vi "Main.vi"() -> ()   [LabVIEW 2022 SP3]
doc: "This Continuous Measurement sample project is based on the Queued Message Handler template.\n\nThe Event Handling Loop generates messages based on user interface actions.\n\nThe Message Handling Loop processes messages generated by the Event Handling Loop, or by other messages. There are also Acquisition and Logging message handling loop subVIs, and a chart updating loop."
uses:
  Settings/Settings.ctl
  Logging/Logging Configuration.ctl
  FiniteMeasurement-DAQmx/controls/Hardware Configuration.ctl
  controls/UI Data.ctl
  controls/UI State.ctl
  Logging/LoggedData.ctl
  support/Message Queue/Enqueue Message (Single).vi
  <vilib>/Utility/error.llb/Error Cluster From Error Code.vi
  <vilib>/ErrorRing/Error Ring.xnode
  Acquisition/Acquisition.lvlib
  Logging/Logging.lvlib
  Settings/Settings.lvlib
  support/User Event - Stop/User Event - Stop.lvlib
  support/Message Queue/Message Queue.lvlib
panel:
  out "FFT- Phase":cluster{dbl, dbl, dbl[]}(graph)
  out "FFT- Mag":cluster{dbl, dbl, dbl[]}(graph)
  in  "Block Size":i32=4096
  in  "Output Settings":bool
  in  "Start Output":bool
  in  "Controller Settings":bool
  in  "Start Controller":bool
  in  "Exit":bool
  in  "Settings":bool
  in  "Start":bool
  in  "Force Trigger":bool
  in  "Stop":bool
  in  "Snapshot":bool
  in  "Analyze":bool
  in  "Clear":bool
  in  "Export":bool
  in  "Save Data":bool
  in  "Load Data":bool
  out "Raw":waveform(dbl)[](graph)
  out "Status":string
  # "Continuous Measurement and Logging (NI-DAQmx)"
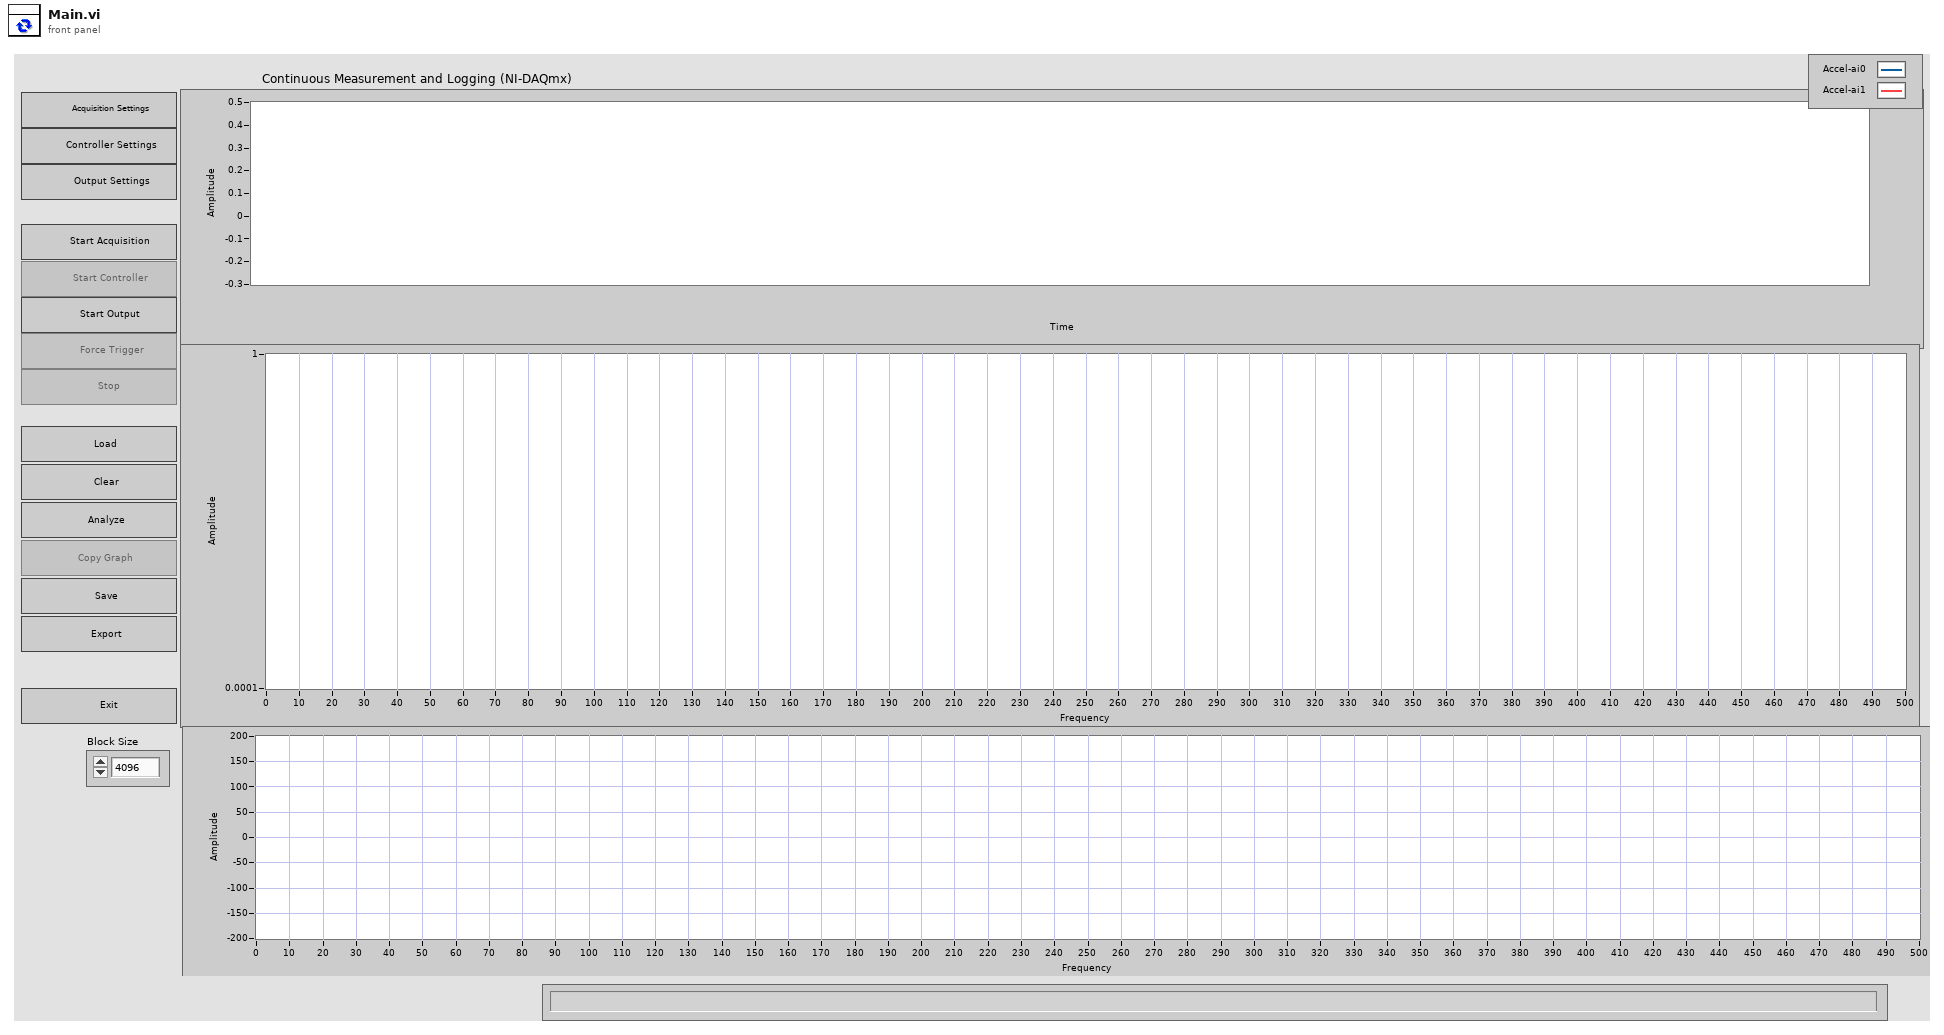
[diagram p1: front panel]
types:
  T1 = typedef "LoggedData.ctl" = cluster{"WaveformArray":waveform(dbl)[], "FFTArray":cluster{dbl, dbl, dbl[]}[]}
  T2 = typedef "UI State.ctl" = enum16{"Idle", "Acquiring and Logging", "Waiting for Exit", "Waiting for Exit (Acq Stopped)", "Waiting for Exit (Log Stopped)", "Waiting for Stop", "Waiting for Stop (Acq Stopped)", "Waiting for Stop (Log Stopped)"}
  T3 = typedef "UI Data.ctl" = cluster{"Start Ref":refnum<vi>, "Trigger Ref":refnum<vi>, "Stop Ref":refnum<vi>, "Settings Ref":refnum<vi>, "Status Ref":refnum<vi>, "Exit Ref":refnum<vi>, "Data Ref":refnum<vi>, "Clear Ref":refnum<vi>, "Load Data Ref":refnum<vi>, "Analyse Ref":refnum<vi>, "Snapshot Ref":refnum<vi>, "Save Data Ref":refnum<vi>, "Export Ref":refnum<vi>, "Output Setting Ref":refnum<vi>, "Start Output Ref":refnum<vi>, "Controller Settings Ref":refnum<vi>, "Start Controller Ref":refnum<vi>}
  T4 = typedef "Settings.lvlib/Settings.ctl" = cluster{"Logging Configuration":T5, "Hardware Configuration":T6}
  T5 = typedef "Logging.lvlib/Logging Configuration.ctl" = cluster{"Log File Base Path":path, "TDMS File Reference":refnum<k34>, "Samples to Save":u32, "Trigger - Time":u32, "Trigger - Threshold":dbl, "Trigger - Channel":u32, "Enable Time Trigger":bool, "Enable Threshold Trigger":bool, "Always Log":bool}
  T6 = typedef "Acquisition.lvlib/Hardware Configuration.ctl" = cluster{"Accel-ai0":bool, "Maximum Input":dbl, "Minimum Input":dbl, "Sample Rate":dbl, "Number of Samples":i32, "Accel-ai1":bool, "DAQmx Task":refnum<k21>}
  T7 = typedef "Message Queue.lvlib/All Message Queues.ctl" = cluster{"UI":refnum<queue>, "Acquisition":refnum<queue>, "Logging":refnum<queue>}
  T8 = enum8{"Enabled", "Disabled", "Disabled and Grayed Out"}
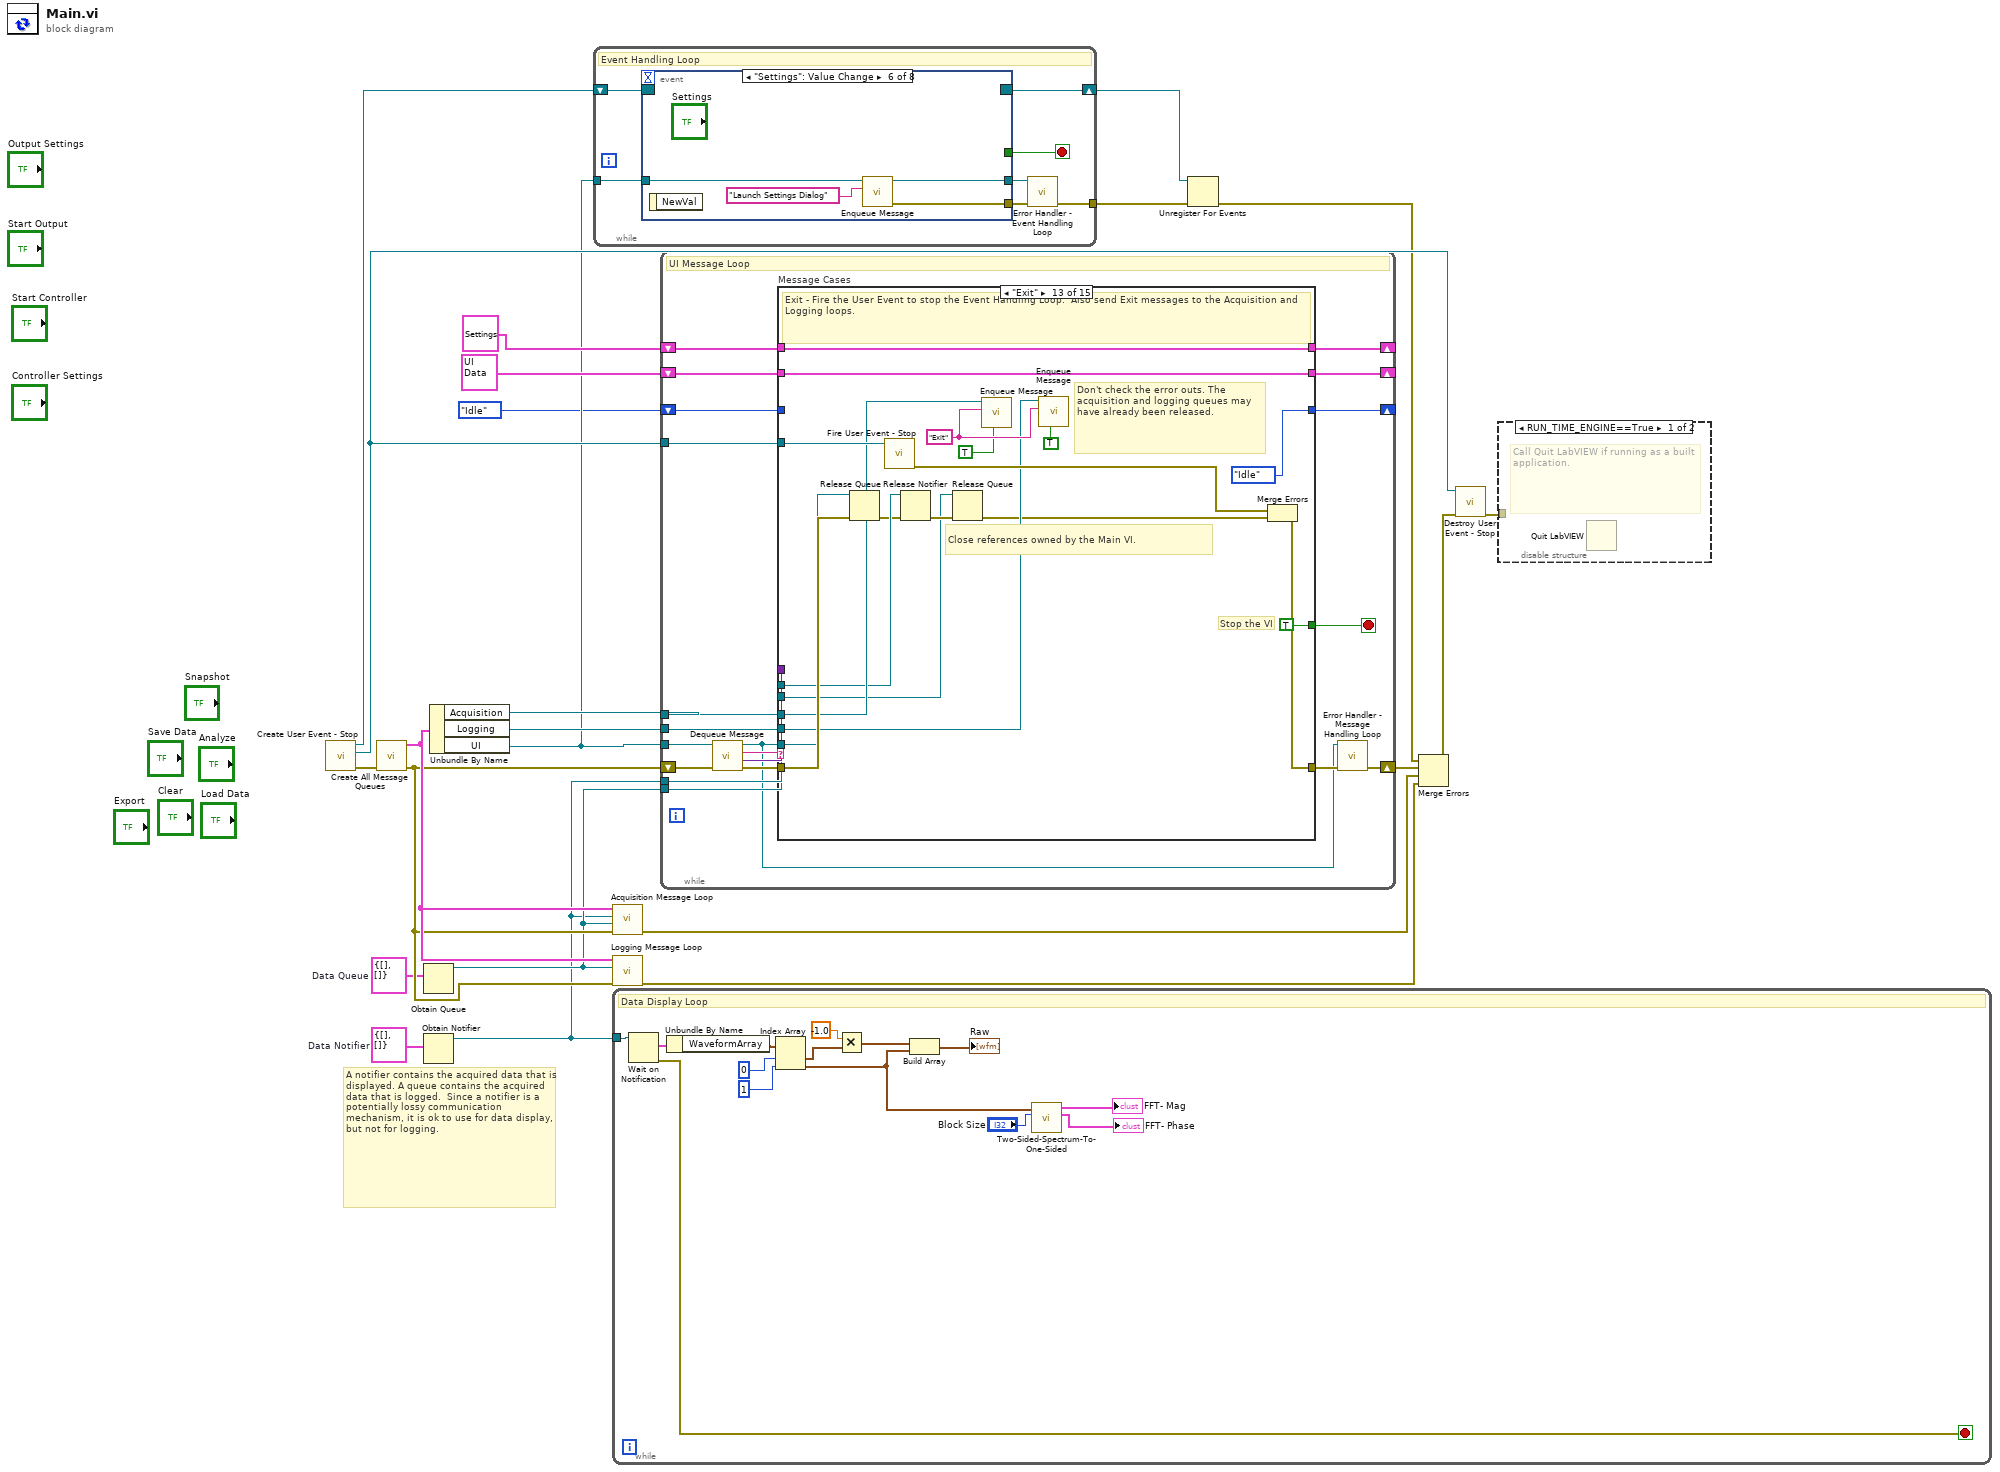
[diagram p0: block diagram]
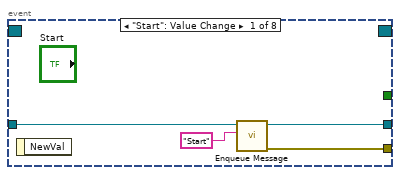
[diagram p3: hidden frame]
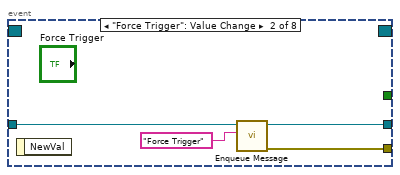
[diagram p4: hidden frame]
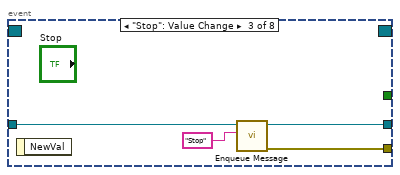
[diagram p5: hidden frame]
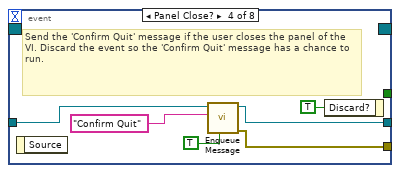
[diagram p6: hidden frame]
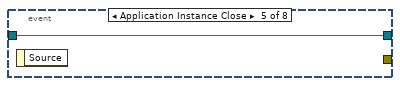
[diagram p7: hidden frame]
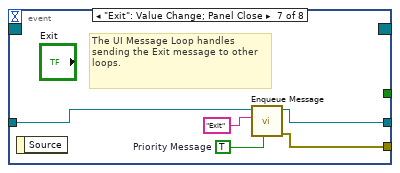
[diagram p8: hidden frame]
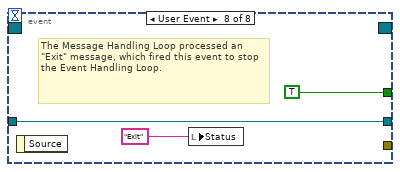
[diagram p9: hidden frame]
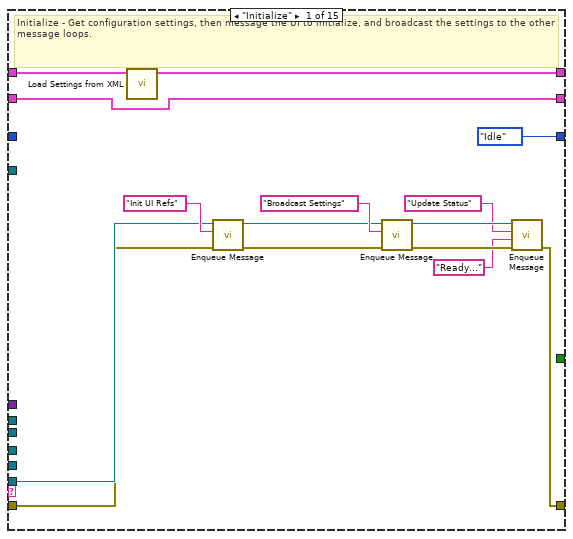
[diagram p10: hidden frame]
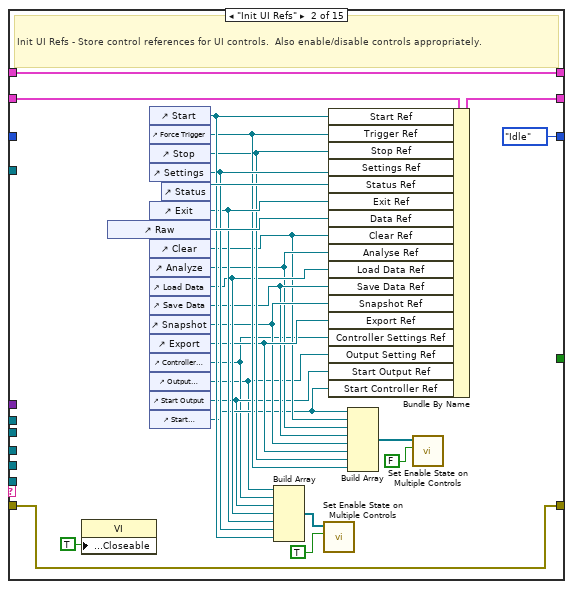
[diagram p11: hidden frame]
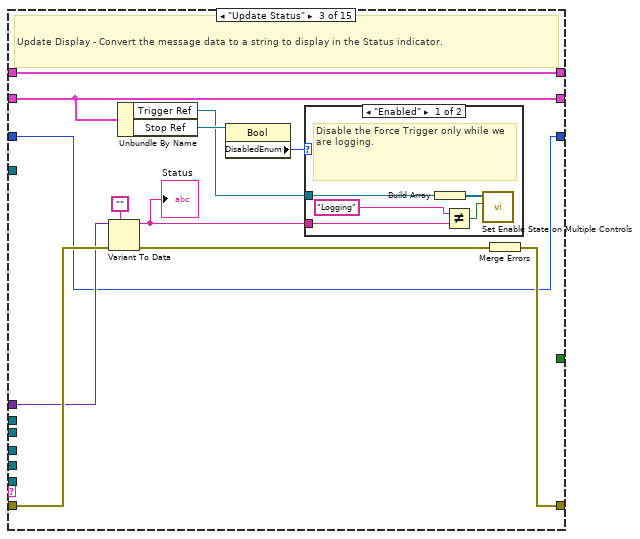
[diagram p12: hidden frame]
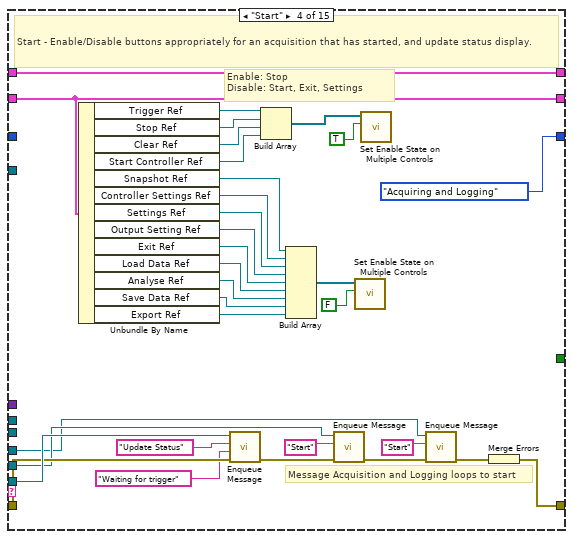
[diagram p14: hidden frame]
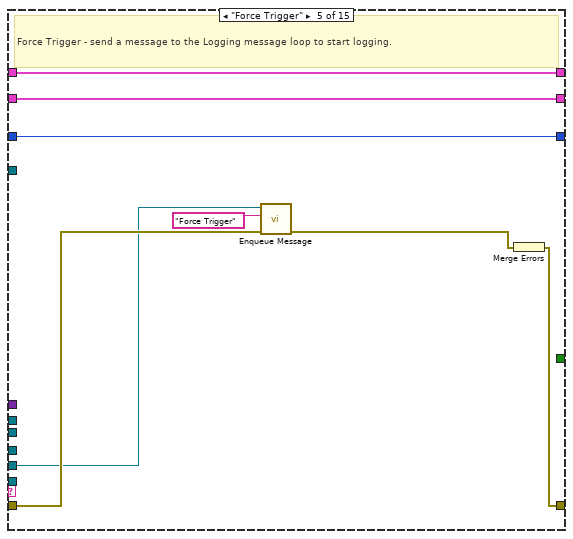
[diagram p15: hidden frame]
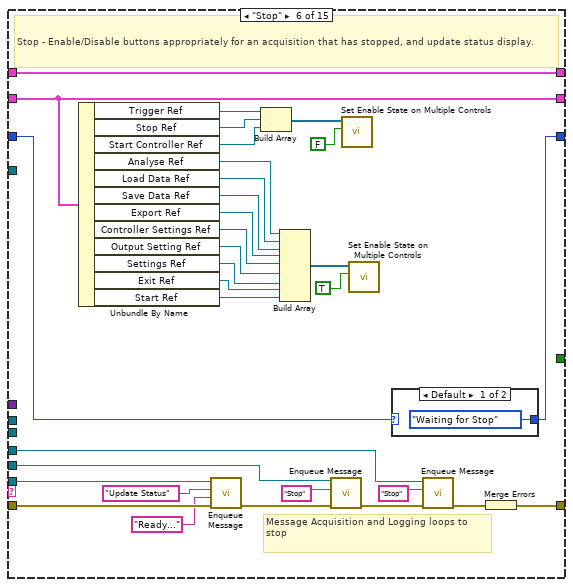
[diagram p16: hidden frame]
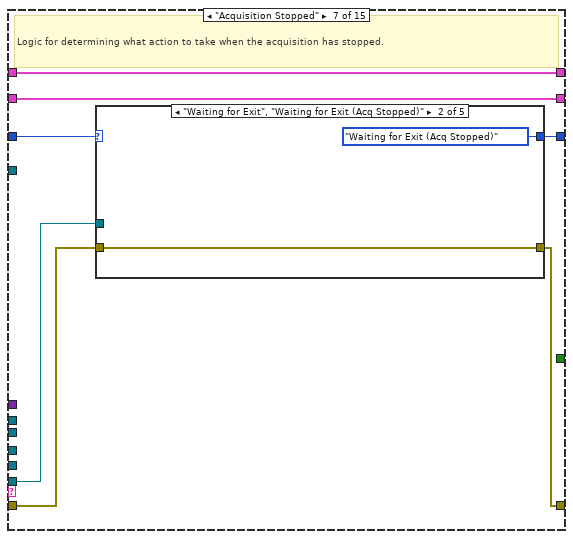
[diagram p18: hidden frame]
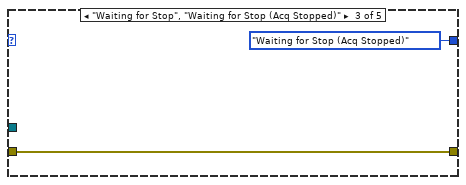
[diagram p20: hidden frame]
diagram:
  w3 = T1 {"WaveformArray"=[], "FFTArray"=[]}  # Data Notifier
  w4 = T1 {"WaveformArray"=[], "FFTArray"=[]}  # Data Queue
  # "A notifier contains the acquired data that is displayed. A queue contains the acquired data that is logged.  Since a notifier is a potentially lossy communication mechanism, it is ok to use for data display, but not for logging."
  n1 = call "Create User Event - Stop.vi"() -> ("error out"=w17:errorcluster, "User Event - Stop"=w19:refnum<user-event>, "Stop Event Registration Refnum"=w20:refnum<event-registration>)  [unwired: 9 in]
  n2 = call "Create All Message Queues.vi"("error in (no error)"=w17) -> ("error out"=w5:errorcluster, "Message Queues out"=w16:T7)  [unwired: 9 in]
  n3 = Obtain Queue(element data type=w4) -> (queue out=w2:refnum<queue>)  [unwired: 4 in, 2 out]
  n4 = Obtain Notifier(notification data type=w3) -> (notifier out=w1:refnum<notifier>)  [unwired: 3 in, 2 out]
  n5 = Unbundle By Name(w16) -> ("Acquisition"=w10:refnum<queue>, "Logging"=w9:refnum<queue>, "UI"=w8:refnum<queue>)
  n6 = while {
    tunnel: w8 -> [w29]
    tunnel: [w24] -> w22
    shift-right: [w28] -> w12
    shift-left: w20 -> [w30]
    stop <- w27 stop-if-true
    # "Event Handling Loop"
    n7 = event shown="[5] \"Settings\": Value Change" {
      selector: w30 -> [_ _ _ _ _ _ _ _]
      dyn-events: [_ _ _ _ _ _ _ _] -> w28
      timeout: _ -> [_ _ _ _ _ _ _ _]
      tunnel: [_ _ _ _ _ _ _ TRUE ("Discard?")] -> w27
      tunnel: w29 -> [w32 w37 w41 w48 w49 w51 w55 w59]
      tunnel: [w34 w36 w40 w43 _ w53 w58 _] -> w25
      tunnel: [w31 w35 w39 w44 w49 w50 w54 w59] -> w26
      event "Start": Value Change {
        n8 = event-data() -> ()  [unwired: 1 in, 1 out]
        n9 = call-poly "Enqueue Message.vi"("Message"="Start", "Message Queue"=w32) -> ("error out"=w34:errorcluster, "dup Message Queue"=w31:refnum<queue>)  [unwired: 8 in]
      }
      event "Force Trigger": Value Change {
        n10 = event-data() -> ()  [unwired: 1 in, 1 out]
        n11 = call-poly "Enqueue Message.vi"("Message"="Force Trigger", "Message Queue"=w37) -> ("error out"=w36:errorcluster, "dup Message Queue"=w35:refnum<queue>)  [unwired: 8 in]
      }
      event "Stop": Value Change {
        n12 = event-data() -> ()  [unwired: 1 in, 1 out]
        n13 = call-poly "Enqueue Message.vi"("Message"="Stop", "Message Queue"=w41) -> ("error out"=w40:errorcluster, "dup Message Queue"=w39:refnum<queue>)  [unwired: 8 in]
      }
      event Panel Close? {
        # "Send the 'Confirm Quit' message if the user closes the panel of the VI. Discard the event so the 'Confirm Quit' message has a chance to run."
        n14 = event-data() -> ()  [unwired: 1 in, 1 out]
        n15 = call-poly "Enqueue Message.vi"("Priority Message? (F)"=TRUE, "Message"="Confirm Quit", "Message Queue"=w48) -> ("error out"=w43:errorcluster, "dup Message Queue"=w44:refnum<queue>)  [unwired: 7 in]
        n16 = event-data("Discard?"=TRUE) -> ()  [unwired: 1 in, 1 out]
      }
      event Application Instance Close {
        n17 = event-data() -> ()  [unwired: 1 in, 1 out]
      }
      event "Settings": Value Change {
        n18 = event-data() -> ()  [unwired: 1 in, 1 out]
        n19 = call-poly "Enqueue Message.vi"("Message"="Launch Settings Dialog", "Message Queue"=w51) -> ("error out"=w53:errorcluster, "dup Message Queue"=w50:refnum<queue>)  [unwired: 8 in]
      }
      event "Exit": Value Change; Panel Close {
        w56 = TRUE  # Priority Message
        # "The UI Message Loop handles sending the Exit message to other loops."
        n20 = event-data() -> ()  [unwired: 1 in, 1 out]
        n21 = call-poly "Enqueue Message.vi"("Priority Message? (F)"=w56, "Message"="Exit", "Message Queue"=w55) -> ("error out"=w58:errorcluster, "dup Message Queue"=w54:refnum<queue>)  [unwired: 7 in]
      }
      event User Event {
        # "The Message Handling Loop processed an \"Exit\" message, which fired this event to stop the Event Handling Loop."
        n22 = event-data() -> ()  [unwired: 1 in, 1 out]
        n23 = local write "Status"("Exit" ("Exit String")) -> ()
      }
    }
    n24 = call "Error Handler - Event Handling Loop.vi"("error in (no error)"=w25, "Message Queue"=w26) -> ("dup error in"=w24:errorcluster)  [unwired: 8 in, 1 out]
  }
  n25 = call "Acquisition Message Loop.vi"("error in (no error)"=w5, "Data Queue"=w2, "Data Notifier"=w1, "Message Queues"=w16) -> ("error out"=w18:errorcluster)  [unwired: 7 in]
  n26 = call "Logging Message Loop.vi"("error in (no error)"=w5, "Data Queue"=w2, "Message Queues"=w16) -> ("error out"=w15:errorcluster)  [unwired: 8 in]
  n27 = while "Data Display Loop" {
    tunnel: w1 -> [w75]
    stop <- w62 stop-if-true
    # "Data Display Loop"
    n28 = Wait on Notification(notifier=w75) -> (notification=w68:T1, error out=w62:errorcluster)  [unwired: 3 in, 2 out]
    n29 = Unbundle By Name(w68) -> ("WaveformArray"=w67:waveform(dbl)[])
    n30 = Index Array(array=w67, index #1=0 ("index"), index #2=1 ("index")) -> (element #1=w70:waveform(dbl), element #2=w66:waveform(dbl))
    n31 = Multiply(x=-1.0, y=w70) -> (x*y=w69:waveform(dbl))
    n32 = Build Array(w69, w66) -> (→"Raw":waveform(dbl)[])
    n33 = call "Two-Sided-Spectrum-To-One-Sided.vi"("Block Size"="Block Size", "waveform"=w66) -> ("FFT- Phase"=→"FFT- Phase":cluster{dbl, dbl, dbl[]}, "FFT- Mag"=→"FFT- Mag":cluster{dbl, dbl, dbl[]})  [unwired: 8 in]
  }
  n34 = while {
    tunnel: w8 -> [w89]
    tunnel: w19 -> [w94]
    shift-right: [w79] -> w23
    shift-left: w5 -> [w93]
    shift-right: [w88] -> _
    shift-left: T4 {"Logging Configuration"={"Log File Base Path"=path "", "TDMS File Reference"=refnum, "Samples to Save"=0, "Trigger - Time"=0, "Trigger - Threshold"=0.0, "Trigger - Channel"=0, "Enable Time Trigger"=FALSE, "Enable Threshold Trigger"=FALSE, "Always Log"=FALSE}, "Hardware Configuration"={"Accel-ai0"=FALSE, "Maximum Input"=0.0, "Minimum Input"=0.0, "Sample Rate"=0.0, "Number of Samples"=0, "Accel-ai1"=FALSE, "DAQmx Task"=""}} ("Settings") -> [w87]
    shift-right: [w85] -> _
    shift-left: T3 {"Start Ref"=refnum, "Trigger Ref"=refnum, "Stop Ref"=refnum, "Settings Ref"=refnum, "Status Ref"=refnum, "Exit Ref"=refnum, "Data Ref"=refnum, "Clear Ref"=refnum, "Load Data Ref"=refnum, "Analyse Ref"=refnum, "Snapshot Ref"=refnum, "Save Data Ref"=refnum, "Export Ref"=refnum, "Output Setting Ref"=refnum, "Start Output Ref"=refnum, "Controller Settings Ref"=refnum, "Start Controller Ref"=refnum} ("Measurement UI Controls") -> [w86]
    tunnel: w10 -> [w84]
    tunnel: w9 -> [w83]
    tunnel: w1 -> [w82]
    tunnel: w2 -> [w81]
    shift-right: [w76] -> _
    shift-left: UI_State."Idle" ("UI State") -> [w77]
    stop <- w95 stop-if-true
    # "UI Message Loop"
    n35 = call "Dequeue Message.vi"("error in (no error)"=w93, "Message Queue"=w89) -> ("error out"=w92:errorcluster, "Message Data"=w90:variant, "Message"=w91:string, "dup Message Queue"=w78:refnum<queue>)  [unwired: 6 in]
    n36 = case "Message Cases" shown="\"Exit\"" w91 {
      selector: w91 -> [_ _ _ _ _ _ _ _ _ _ _ _ _ _ w371]
      tunnel: w78 -> [w100 _ _ w185 _ w225 w229 w254 _ w296 w311 w321 w354 _ _]
      tunnel: w92 -> [w99 w137 w148 w184 w191 w224 w231 w256 w284 w298 w315 w320 w362 w369 _]
      tunnel: [w106 w137 w149 w186 w194 w226 w230 w255 w290 w293 w306 w319 w363 w368 w372] -> w80
      tunnel: [_ _ _ _ _ _ _ _ _ _ _ _ TRUE _ _] -> w95
      tunnel: w90 -> [_ _ w147 _ _ _ _ _ _ _ w314 _ _ _ _]
      tunnel: w94 -> [_ _ _ _ _ _ _ _ _ _ _ _ w361 _ _]
      tunnel: [w109 w136 w144 w183 w193 w223 w235 w260 w288 w295 w317 w324 w359 w367 w374] -> w88
      tunnel: w87 -> [w110 w136 w144 w183 w193 w223 w235 w260 w288 w299 w317 w324 w359 w367 w374]
      tunnel: w86 -> [w102 w135 w143 w180 w192 w220 w234 w259 w282 w292 w316 w323 w357 w366 w373]
      tunnel: [w102 w134 w143 w180 w192 w220 w234 w259 w282 w292 w316 w323 w357 w366 w373] -> w85
      tunnel: w84 -> [_ _ _ w170 _ w210 _ _ w281 _ _ _ w356 _ _]
      tunnel: w83 -> [_ _ _ w173 w188 w213 _ _ w280 _ _ _ w355 _ _]
      tunnel: w82 -> [_ _ _ _ _ _ _ _ _ _ _ _ w353 _ _]
      tunnel: w81 -> [_ _ _ _ _ _ _ _ _ _ _ _ w349 _ _]
      tunnel: w77 -> [_ _ w138 _ w187 w206 w233 w258 w279 w291 w305 w322 _ w365 w370]
      tunnel: [UI_State."Idle" ("UI State") UI_State."Idle" ("UI State") w138 UI_State."Acquiring and Logging" ("UI State") w187 w205 w232 w257 w279 w291 w305 w318 UI_State."Idle" ("UI State") w365 w370] -> w76
      frame "Initialize" {
        # "Initialize - Get configuration settings, then message the UI to initialize, and broadcast the settings to the other message loops."
        n37 = call "Load Settings from XML.vi"("Settings in"=w110) -> ("Settings out"=w109:T4)  [unwired: 9 in, 1 out]
        n38 = call-poly "Enqueue Message.vi"("error in (no error)"=w99, "Message"="Init UI Refs", "Message Queue"=w100) -> ("error out"=w97:errorcluster, "dup Message Queue"=w98:refnum<queue>)  [unwired: 7 in]
        n39 = call-poly "Enqueue Message.vi"("error in (no error)"=w97, "Message"="Broadcast Settings", "Message Queue"=w98) -> ("error out"=w108:errorcluster, "dup Message Queue"=w107:refnum<queue>)  [unwired: 7 in]
        n40 = call-poly "Enqueue Message.vi"("error in (no error)"=w108, "Message Data"="Ready..." ("Ready..."), "Message"="Update Status", "Message Queue"=w107) -> ("error out"=w106:errorcluster)  [unwired: 6 in, 1 out]
      }
      frame "Init UI Refs" {
        # "Init UI Refs - Store control references for UI controls.  Also enable/disable controls appropriately."
        n41 = property class="VI"("Front Panel.Closeable"=TRUE ("Front Panel Window:Closeable")) -> ()  [unwired: 2 in, 2 out]
        n42 = control-ref of="Raw"() -> (w130:refnum<vi>)
        n43 = control-ref of="Start"() -> (w129:refnum<vi>)
        n44 = control-ref of="Force Trigger"() -> (w124:refnum<vi>)
        n45 = control-ref of="Stop"() -> (w123:refnum<vi>)
        n46 = control-ref of="Settings"() -> (w126:refnum<vi>)
        n47 = control-ref of="Exit"() -> (w125:refnum<vi>)
        n48 = control-ref of="Clear"() -> (w115:refnum<vi>)
        n49 = control-ref of="Analyze"() -> (w116:refnum<vi>)
        n50 = control-ref of="Load Data"() -> (w120:refnum<vi>)
        n51 = control-ref of="Save Data"() -> (w117:refnum<vi>)
        n52 = control-ref of="Snapshot"() -> (w118:refnum<vi>)
        n53 = control-ref of="Export"() -> (w119:refnum<vi>)
        n54 = control-ref of="Controller Settings"() -> (w112:refnum<vi>)
        n55 = control-ref of="Output Settings"() -> (w111:refnum<vi>)
        n56 = control-ref of="Start Output"() -> (w113:refnum<vi>)
        n57 = control-ref of="Start Controller"() -> (w114:refnum<vi>)
        n58 = control-ref of="Status"() -> (w131:refnum<vi>)
        n59 = Build Array(w111, w112, w113, w120, w125, w126, w129) -> (w128:refnum<vi>[])
        n60 = call "Set Enable State on Multiple Controls.vi"("Enable?"=TRUE, "Controls"=w128) -> ()  [unwired: 10 in]
        n61 = Bundle By Name(cluster=w135, "Start Ref"=w129, "Trigger Ref"=w124, "Stop Ref"=w123, "Settings Ref"=w126, "Status Ref"=w131, "Exit Ref"=w125, "Data Ref"=w130, "Clear Ref"=w115, "Analyse Ref"=w116, "Load Data Ref"=w120, "Save Data Ref"=w117, "Snapshot Ref"=w118, "Export Ref"=w119, "Controller Settings Ref"=w112, "Output Setting Ref"=w111, "Start Output Ref"=w113, "Start Controller Ref"=w114) -> (w134:T3)
        n62 = Build Array(w114, w115, w116, w117, w118, w119, w123, w124) -> (w122:refnum<vi>[])
        n63 = call "Set Enable State on Multiple Controls.vi"("Enable?"=FALSE, "Controls"=w122) -> ()  [unwired: 10 in]
      }
      frame "Update Status" {
        # "Update Display - Convert the message data to a string to display in the Status indicator."
        n64 = Variant To Data(error in=w148, type="", Variant=w147) -> (data=w140:string, error out=w145:errorcluster)
        "Status" <- w140
        n65 = Unbundle By Name(w143) -> ("Trigger Ref"=w139:refnum<vi>, "Stop Ref"=w142:refnum<vi>)
        n66 = property class="Bool"(reference=w142) -> ("DisabledEnum"=w141:T8)  [unwired: 1 in, 2 out]
        n67 = case shown="\"Enabled\"" w141 {
          tunnel: w140 -> [w152 _]
          tunnel: w139 -> [w153 _]
          frame "Enabled" {
            # "Disable the Force Trigger only while we are logging."
            n68 = Build Array(w153) -> (w154:refnum<vi>[])
            n69 = Not Equal?(x="Logging" ("Logging"), y=w152) -> (x != y?=w150:bool)
            n70 = call "Set Enable State on Multiple Controls.vi"("Enable?"=w150, "Controls"=w154) -> ()  [unwired: 10 in]
          }
          frame "Disabled", Default {
          }
        }
        n71 = Merge Errors(w145) -> (w149:errorcluster)
      }
      frame "Start" {
        # "Message Acquisition and Logging loops to start"
        # "Enable: Stop\nDisable: Start, Exit, Settings"
        # "Start - Enable/Disable buttons appropriately for an acquisition that has started, and update status display."
        n72 = Unbundle By Name(w180) -> ("Trigger Ref"=w167:refnum<vi>, "Stop Ref"=w168:refnum<vi>, "Clear Ref"=w165:refnum<vi>, "Start Controller Ref"=w164:refnum<vi>, "Snapshot Ref"=w155:refnum<vi>, "Controller Settings Ref"=w156:refnum<vi>, "Settings Ref"=w157:refnum<vi>, "Output Setting Ref"=w158:refnum<vi>, "Exit Ref"=w159:refnum<vi>, "Load Data Ref"=w160:refnum<vi>, "Analyse Ref"=w161:refnum<vi>, "Save Data Ref"=w162:refnum<vi>, "Export Ref"=w163:refnum<vi>)
        n73 = call-poly "Enqueue Message.vi"("error in (no error)"=w184, "Message Data"="Waiting for trigger" ("Waiting for trigger"), "Message"="Update Status", "Message Queue"=w185) -> ("error out"=w175:errorcluster)  [unwired: 6 in, 1 out]
        n74 = Build Array(w167, w168, w165, w164) -> (w177:refnum<vi>[])
        n75 = Build Array(w155, w156, w157, w158, w159, w160, w161, w162, w163) -> (w178:refnum<vi>[])
        n76 = call-poly "Enqueue Message.vi"("error in (no error)"=w175, "Message"="Start", "Message Queue"=w173) -> ("error out"=w172:errorcluster)  [unwired: 7 in, 1 out]
        n77 = call "Set Enable State on Multiple Controls.vi"("Enable?"=FALSE, "Controls"=w178) -> ()  [unwired: 10 in]
        n78 = call "Set Enable State on Multiple Controls.vi"("Enable?"=TRUE, "Controls"=w177) -> ()  [unwired: 10 in]
        n79 = call-poly "Enqueue Message.vi"("error in (no error)"=w172, "Message"="Start", "Message Queue"=w170) -> ("error out"=w171:errorcluster)  [unwired: 7 in, 1 out]
        n80 = Merge Errors(w171) -> (w186:errorcluster)
      }
      frame "Force Trigger" {
        # "Force Trigger - send a message to the Logging message loop to start logging."
        n81 = call-poly "Enqueue Message.vi"("error in (no error)"=w191, "Message"="Force Trigger", "Message Queue"=w188) -> ("error out"=w190:errorcluster)  [unwired: 7 in, 1 out]
        n82 = Merge Errors(w190) -> (w194:errorcluster)
      }
      frame "Stop" {
        # "Message Acquisition and Logging loops to stop"
        # "Stop - Enable/Disable buttons appropriately for an acquisition that has stopped, and update status display."
        n83 = Unbundle By Name(w220) -> ("Trigger Ref"=w207:refnum<vi>, "Stop Ref"=w208:refnum<vi>, "Start Controller Ref"=w204:refnum<vi>, "Analyse Ref"=w195:refnum<vi>, "Load Data Ref"=w196:refnum<vi>, "Save Data Ref"=w197:refnum<vi>, "Export Ref"=w198:refnum<vi>, "Controller Settings Ref"=w199:refnum<vi>, "Output Setting Ref"=w200:refnum<vi>, "Settings Ref"=w201:refnum<vi>, "Exit Ref"=w202:refnum<vi>, "Start Ref"=w203:refnum<vi>)
        n84 = call-poly "Enqueue Message.vi"("error in (no error)"=w224, "Message Data"="Ready..." ("Ready..."), "Message"="Update Status", "Message Queue"=w225) -> ("error out"=w215:errorcluster)  [unwired: 6 in, 1 out]
        n85 = Build Array(w207, w208, w204) -> (w217:refnum<vi>[])
        n86 = Build Array(w195, w196, w197, w198, w199, w200, w201, w202, w203) -> (w218:refnum<vi>[])
        n87 = call-poly "Enqueue Message.vi"("error in (no error)"=w215, "Message"="Stop", "Message Queue"=w213) -> ("error out"=w212:errorcluster)  [unwired: 7 in, 1 out]
        n88 = call "Set Enable State on Multiple Controls.vi"("Enable?"=FALSE, "Controls"=w217) -> ()  [unwired: 10 in]
        n89 = call "Set Enable State on Multiple Controls.vi"("Enable?"=TRUE, "Controls"=w218) -> ()  [unwired: 10 in]
        n90 = case shown="Default" w206 {
          selector: w206 -> [_ w228]
          tunnel: [UI_State."Waiting for Stop" ("UI State") w228] -> w205
          frame Default {
          }
          frame "Waiting for Exit" {
          }
        }
        n91 = call-poly "Enqueue Message.vi"("error in (no error)"=w212, "Message"="Stop", "Message Queue"=w210) -> ("error out"=w211:errorcluster)  [unwired: 7 in, 1 out]
        n92 = Merge Errors(w211) -> (w226:errorcluster)
      }
      frame "Acquisition Stopped" {
        # "Logic for determining what action to take when the acquisition has stopped."
        n93 = case shown="\"Waiting for Exit\", \"Waiting for Exit (Acq Stopped)\"" w233 {
          selector: w233 -> [w237 _ _ _ _]
          tunnel: [w237 UI_State."Waiting for Exit (Acq Stopped)" ("UI State") UI_State."Waiting for Stop (Acq Stopped)" ("UI State") UI_State."Idle" ("UI State") UI_State."Idle" ("UI State")] -> w232
          tunnel: w231 -> [w236 w238 w240 w246 w252]
          tunnel: [w236 w238 w240 w245 w251] -> w230
          tunnel: w229 -> [_ _ _ w244 w250]
          frame Default {
          }
          frame "Waiting for Exit", "Waiting for Exit (Acq Stopped)" {
          }
          frame "Waiting for Stop", "Waiting for Stop (Acq Stopped)" {
          }
          frame "Waiting for Exit (Log Stopped)" {
            # "If we are waiting to exit, and the logging has already stopped, then the \"Acquisition Stopped\" message indicates that it is time to exit."
            n94 = call-poly "Enqueue Message.vi"("Priority Message? (F)"=TRUE, "error in (no error)"=w246, "Message"="Exit", "Message Queue"=w244) -> ("error out"=w245:errorcluster)  [unwired: 6 in, 1 out]
          }
          frame "Waiting for Stop (Log Stopped)" {
            # "If we are waiting to stop, and the logging has already stopped, then the \"Acquisition Stopped\" message indicates that it is time to stop."
            n95 = call-poly "Enqueue Message.vi"("error in (no error)"=w252, "Message Data"="Ready..." ("Message"), "Message"="Update Status", "Message Queue"=w250) -> ("error out"=w251:errorcluster)  [unwired: 6 in, 1 out]
          }
        }
      }
      frame "Logging Stopped" {
        # "Logic for determining what action to take when the logging has stopped."
        n96 = case shown="\"Waiting for Stop (Acq Stopped)\"" w258 {
          selector: w258 -> [w262 _ _ _ _]
          tunnel: [w262 UI_State."Waiting for Exit (Log Stopped)" ("UI State") UI_State."Waiting for Stop (Log Stopped)" ("UI State") UI_State."Idle" ("UI State") UI_State."Idle" ("UI State")] -> w257
          tunnel: w256 -> [w261 w263 w265 w271 w277]
          tunnel: [w261 w263 w265 w270 w276] -> w255
          tunnel: w254 -> [_ _ _ w269 w275]
          frame Default {
          }
          frame "Waiting for Exit", "Waiting for Exit (Log Stopped)" {
          }
          frame "Waiting for Stop", "Waiting for Stop (Log Stopped)" {
          }
          frame "Waiting for Exit (Acq Stopped)" {
            # "If we are waiting to exit, and the acquisition has already stopped, then the \"Logging Stopped\" message indicates that it is time to exit."
            n97 = call-poly "Enqueue Message.vi"("Priority Message? (F)"=TRUE, "error in (no error)"=w271, "Message"="Exit", "Message Queue"=w269) -> ("error out"=w270:errorcluster)  [unwired: 6 in, 1 out]
          }
          frame "Waiting for Stop (Acq Stopped)" {
            # "If we are waiting to stop, and the acquisition has already stopped, then the \"Logging Stopped\" message indicates that it is time to stop."
            n98 = call-poly "Enqueue Message.vi"("error in (no error)"=w277, "Message Data"="Ready..." ("Message"), "Message"="Update Status", "Message Queue"=w275) -> ("error out"=w276:errorcluster)  [unwired: 6 in, 1 out]
          }
        }
      }
      frame "Broadcast settings" {
        w283 = "Update Settings" ("Message")
        # "Send the 'Update Settings' message to the Logging and Acquisition message loops."
        n99 = Unbundle By Name(w288) -> ("Hardware Configuration"=w287:T6, "Logging Configuration"=w286:T5)
        n100 = call-poly "Enqueue Message.vi"("Message Data"=w287, "Message"=w283, "Message Queue"=w281) -> ("error out"=w289:errorcluster)  [unwired: 7 in, 1 out]
        n101 = call-poly "Enqueue Message.vi"("error in (no error)"=w289, "Message Data"=w286, "Message"=w283, "Message Queue"=w280) -> ("error out"=w285:errorcluster)  [unwired: 6 in, 1 out]
        n102 = Merge Errors(w285, w284) -> (w290:errorcluster)
      }
      frame "Launch Settings Dialog" {
        # "Launch the Settings Dialog when the user clicks the 'Settings' button."
        n103 = call "Settings Dialog.vi"("error in (no error)"=w298, "Settings in"=w299) -> ("error out"=w294:errorcluster, "Cancelled?"=w297:bool, "Settings Out"=w295:T4)  [unwired: 6 in, 1 out]
        n104 = case shown="False" w297 {
          tunnel: w296 -> [w303 _]
          tunnel: w294 -> [w302 w304]
          tunnel: [w301 w304] -> w293
          frame False {
            n105 = call-poly "Enqueue Message.vi"("error in (no error)"=w302, "Message"="Broadcast Settings", "Message Queue"=w303) -> ("error out"=w301:errorcluster)  [unwired: 7 in, 1 out]
          }
          frame True {
          }
        }
      }
      frame "Error" {
        # "Error - Check the error message data and respond accordingly. This message is sent by the \"Error Handler\" VIs at the end of each loop in this application."
        n106 = Variant To Data(error in=w315, type=errorcluster {"status"=FALSE, "code"=0, "source"=""} ("error out"), Variant=w314) -> (data=w312:errorcluster, error out=w308:errorcluster)
        n107 = call <vilib>:"Simple Error Handler.vi"("error in (no error)"=w312) -> ()  [unwired: 4 in, 5 out]
        n108 = call-poly "Enqueue Message.vi"("Priority Message? (F)"=TRUE, "Message"="Exit", "Message Queue"=w311) -> ("error out"=w307:errorcluster)  [unwired: 7 in, 1 out]
        n109 = Merge Errors(w307, w308) -> (w306:errorcluster)
      }
      frame "Confirm Quit" {
        # "Confirm Quit - Message that can confirm whether or not the user wants to exit the application."
        n110 = case shown="\"Acquiring and Logging\"" w322 {
          tunnel: w321 -> [w329 w335]
          tunnel: w320 -> [w328 w333]
          tunnel: [w325 w332] -> w319
          tunnel: [UI_State."Idle" ("UI State") w331] -> w318
          frame Default {
            # "If 'Confirm Quit' comes in while the system is idle, there is no need for a confirmation message."
            n111 = call-poly "Enqueue Message.vi"("Priority Message? (F)"=TRUE, "error in (no error)"=w328, "Message"="Exit", "Message Queue"=w329) -> ("error out"=w325:errorcluster)  [unwired: 6 in, 1 out]
          }
          frame "Acquiring and Logging" {
            n112 = Two Button Dialog(message="Are you sure you want to quit while the acquisition is running?" ("Confirm Quit Message"), 1:"No" ("No"), 2:"Yes" ("Yes")) -> (T button?=w334:bool)
            n113 = case shown="True" w334 {
              tunnel: w335 -> [_ w345]
              tunnel: w333 -> [w339 w344]
              tunnel: [w339 w343] -> w332
              tunnel: [UI_State."Acquiring and Logging" ("UI State") UI_State."Waiting for Exit" ("UI State")] -> w331
              frame False {
                # "User did not want to quit."
              }
              frame True {
                n114 = call-poly "Enqueue Message.vi"("error in (no error)"=w344, "Message"="Stop", "Message Queue"=w345) -> ("error out"=w343:errorcluster)  [unwired: 7 in, 1 out]
              }
            }
          }
        }
      }
      frame "Exit" {
        w358 = "Exit" ("Message")
        # "Don't check the error outs. The acquisition and logging queues may have already been released."
        # "Close references owned by the Main VI."
        # "Stop the VI"
        # "Exit - Fire the User Event to stop the Event Handling Loop.  Also send Exit messages to the Acquisition and Logging loops."
        n115 = Release Queue(queue=w354, error in (no error)=w362) -> (error out=w352:errorcluster)  [unwired: 1 in, 2 out]
        n116 = call "Fire User Event - Stop.vi"("User Event - Stop"=w361) -> ("error out"=w360:errorcluster)  [unwired: 10 in]
        n117 = Release Notifier(notifier=w353, error in (no error)=w352) -> (error out=w351:errorcluster)  [unwired: 1 in, 2 out]
        n118 = Release Queue(queue=w349, error in (no error)=w351) -> (error out=w350:errorcluster)  [unwired: 1 in, 2 out]
        n119 = call-poly "Enqueue Message.vi"("Priority Message? (F)"=TRUE, "Message"=w358, "Message Queue"=w356) -> ()  [unwired: 7 in, 2 out]
        n120 = call-poly "Enqueue Message.vi"("Priority Message? (F)"=TRUE, "Message"=w358, "Message Queue"=w355) -> ()  [unwired: 7 in, 2 out]
        n121 = Merge Errors(w360, w350) -> (w363:errorcluster)
      }
      frame "---Copy This Frame---" {
        # "Duplicate this frame when creating new messages.  Change this comment in the duplicated frame to describe this message."
        n122 = Merge Errors(w369) -> (w368:errorcluster)
      }
      frame Default {
        # "'Default' case only runs if there is a message that isn't defined in any of the other cases.  Output a programming error."
        n123 = xnode "Error Ring"("parameter 0"=w371) -> ("error out"=w372:errorcluster)
      }
    }
    n124 = call "Error Handler - Message Handling Loop.vi"("error in (no error)"=w80, "Message Queue"=w78) -> ("dup error in"=w79:errorcluster)  [unwired: 8 in, 1 out]
  }
  n125 = Unregister For Events(event registration refnum=w12, error in=w22) -> (error out=w13:errorcluster)
  n126 = Merge Errors(w13, w23, w18, w15) -> (w21:errorcluster)
  n127 = call "Destroy User Event - Stop.vi"("error in (no error)"=w21, "User Event - Stop"=w19) -> ("error out"=w7:errorcluster)  [unwired: 9 in]
  n128 = disable-structure shown="RUN_TIME_ENGINE==True" {
    disable-tunnel: w7 -> [_ _]
    frame condition #0 {
      # "Call Quit LabVIEW if running as a built application."
      n129 = Quit LabVIEW() -> ()  [unwired: 1 in]
    }
    frame condition #1 (active) {
    }
  }
